vi "Exctracted AVI1-2 code.vi"   [LabVIEW 2017]
types:
  T1 = typedef "IMAQ AVI2 Refnum.ctl" = refnum<k20>
  T2 = typedef "IMAQ Image.ctl" = refnum<image>
  T3 = typedef "AviRefnum.ctl" = refnum<k1>
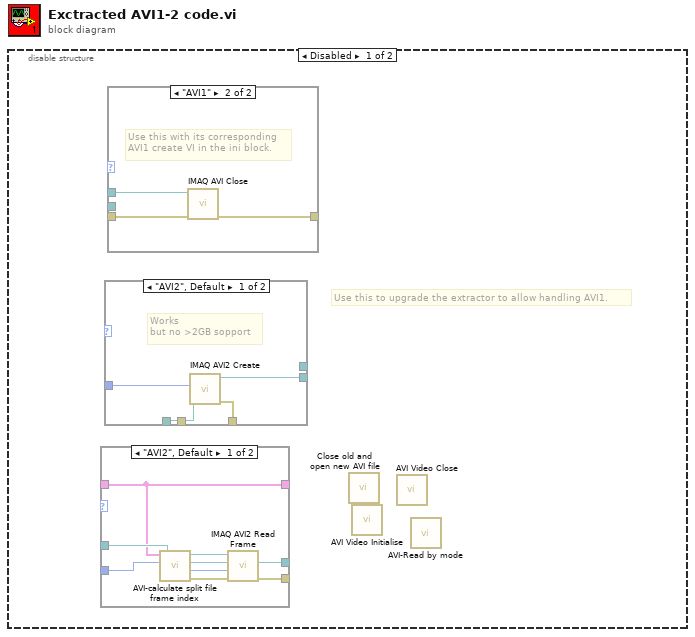
[diagram p0: block diagram]
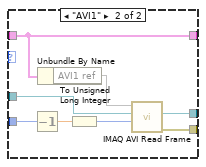
[diagram p2: hidden frame]
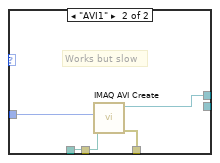
[diagram p3: hidden frame]
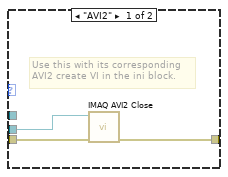
[diagram p4: hidden frame]
diagram:
  n1 = disable-structure shown="Disabled" {
    frame Disabled {
      # "Use this to upgrade the extractor to allow handling AVI1."
      n2 = case shown="\"AVI2\", Default" {
        selector: _ -> [_ _]
        tunnel: [w6 w16] -> _
        tunnel: [w8 w15] -> _
        tunnel: _ -> [w1 w9]
        tunnel: _ -> [w7 w14]
        tunnel: [w1 w9] -> _
        tunnel: _ -> [w2 w11]
        frame "AVI2", Default {
          n3 = call "AVI-calculate split file frame index.vi"("Frame number (unity-based) in"=w2, "AVI modes refs"=w1) -> ("error out"=w4:errorcluster, "Index of frame in split file"=w5:u32, "AVI2 split file ref"=w3:T1)  [unwired: 6 in, 1 out]
          n4 = call "IMAQ AVI2 Read Frame"("error in (no error)"=w4, "Frame Number"=w5, "Image"=w7, "AVI Refnum"=w3) -> ("error out"=w6:errorcluster, "Image Out"=w8:T2)  [unwired: 5 in, 1 out]
        }
        frame "AVI1" {
          n5 = Decrement(x=w11) -> (x-1=w10:dbl)
          n6 = Unbundle By Name(w9) -> ("AVI1 ref"=w13)
          n7 = To Unsigned Long Integer(number=w10) -> (unsigned 32bit integer=w12:u32)
          n8 = call "IMAQ AVI Read Frame"("Frame Number"=w12, "Image"=w14, "Avi Refnum"=w13) -> ("error out"=w16:errorcluster, "Image Out"=w15:T2)  [unwired: 5 in, 2 out]
        }
      }
      n9 = case shown="\"AVI2\", Default" {
        selector: _ -> [_ _]
        tunnel: _ -> [w21 w26]
        tunnel: _ -> [w20 w25]
        tunnel: _ -> [w19 w24]
        tunnel: [w18 w23] -> _
        tunnel: [w17 _] -> _
        tunnel: [_ w22] -> _
        frame "AVI2", Default {
          # "Works\nbut no >2GB sopport"
          n10 = call "IMAQ AVI2 Create"("error in (no error)"=w19, "Frames Per Second"=w21, "AVI Path"=w20) -> ("error out"=w18:errorcluster, "AVI Refnum"=w17:T1)  [unwired: 7 in]
        }
        frame "AVI1" {
          # "Works but slow"
          n11 = call "IMAQ AVI Create"("error in (no error)"=w24, "Frames Per Second"=w26, "AVI Path"=w25) -> ("error out"=w23:errorcluster, "Avi Refnum"=w22:T3)  [unwired: 7 in]
        }
      }
      n12 = case shown="\"AVI1\"" {
        selector: _ -> [_ _]
        tunnel: _ -> [w29 _]
        tunnel: [w28 w32] -> _
        tunnel: _ -> [w27 w31]
        tunnel: _ -> [_ w30]
        frame "AVI2" {
          # "Use this with its corresponding\nAVI2 create VI in the ini block."
          n13 = call "IMAQ AVI2 Close"("error in (no error)"=w27, "AVI Refnum"=w29) -> ("error out"=w28:errorcluster)  [unwired: 9 in]
        }
        frame "AVI1" {
          # "Use this with its corresponding\nAVI1 create VI in the ini block."
          n14 = call "IMAQ AVI Close"("error in (no error)"=w31, "Avi Refnum"=w30) -> ("error out"=w32:errorcluster)  [unwired: 9 in]
        }
      }
      n15 = call "Close old and open new AVI file.vi"() -> ()  [unwired: 7 in, 5 out]
      n16 = call "AVI Video Initialise.vi"() -> ()  [unwired: 11 in, 1 out]
      n17 = call "AVI Video Close.vi"() -> ()  [unwired: 11 in, 1 out]
      n18 = call "AVI-Read by mode.vi"() -> ()  [unwired: 9 in, 3 out]
    }
    frame Enabled {
    }
  }
